vi "lcm.vi"(10 "DAC Frequency":i32=1200, 11 "Frequency":i32=300) -> (3 "Number of Points":i32)   [LabVIEW 2016]
uses:
  <vilib>/gmath/NI_Gmath.lvlib
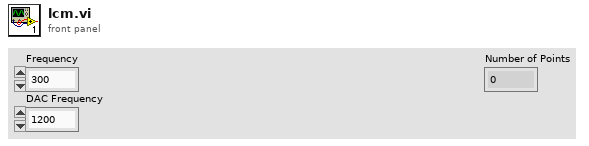
[diagram p1: front panel]
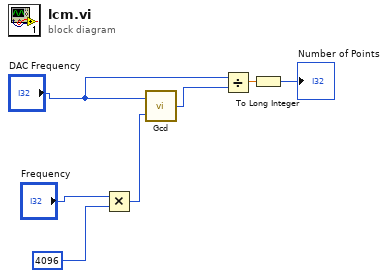
[diagram p0: block diagram]
diagram:
  n1 = Multiply(x="Frequency", y=4096) -> (x*y=w4:i32)
  n2 = call <vilib>:"Gcd.vi"("y"=w4, "x"="DAC Frequency") -> ("gcd(x,y)"=w3:i32)
  n3 = Divide(x="DAC Frequency", y=w3) -> (x/y=w1:dbl)
  n4 = To Long Integer(number=w1) -> (32bit integer=→"Number of Points":i32)
